vi "SIM_Drive_Gyro_EXECUTE.vi"(6 "FPGA_Time_Seconds":dbl, 8 "error in (no error)":errorcluster, 11 "ModuleStates":T1[](array[typedef]) {"Angle"."SIN" format="%13.4f"; "Angle"."COS" format="%13.4f"; "Angle"."VALUE" format="%13.4f"}) -> (0 "error out":errorcluster, 3 "GyroYawDegrees":dbl)   [LabVIEW 2023]
uses:
  <vilib>/Rock Robotics/WPI/ThirdParty/JAS_Junk/TrajLib/TypeDef/SWERVE_DRIVE_MODULE_STATE.ctl
  <vilib>/Rock Robotics/WPI/ThirdParty/JAS_Junk/TrajLib/TypeDef/ROTATION2D.ctl
  SIM_Drive_Globals.vi
  <vilib>/Rock Robotics/WPI/ThirdParty/JAS_Junk/TrajLib/Trajectory_Library.lvlib
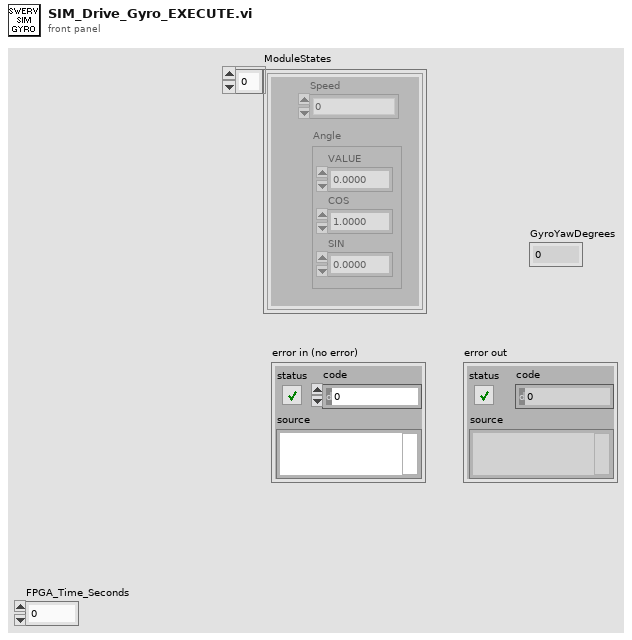
[diagram p1: front panel]
types:
  T1 = typedef "Trajectory_Library.lvlib/SWERVE_DRIVE_MODULE_STATE.ctl" = cluster{"Speed":dbl, "Angle":T2}
  T2 = typedef "Trajectory_Library.lvlib/ROTATION2D.ctl" = cluster{"VALUE":dbl, "COS":dbl, "SIN":dbl}
  T3 = typedef "Trajectory_Library.lvlib/SWERVE_DRIVE_KINEMATICS.ctl" = cluster{"NumModules":i32, "InverseKinematics":T4, "ForwardKinematics":T4, "Modules":T5[], "PrevCoR":T5, "SavedModuleStates":T1[]}
  T4 = typedef "NI_Matrix.lvlib/RealMatrix.ctl" = dbl[][]
  T5 = typedef "Trajectory_Library.lvlib/TRANSLATION2D.ctl" = cluster{"X":dbl, "Y":dbl}
  T6 = typedef "Trajectory_Library.lvlib/CHASSIS_SPEEDS.ctl" = cluster{"vX":dbl, "vY":dbl, "vOmega":dbl}
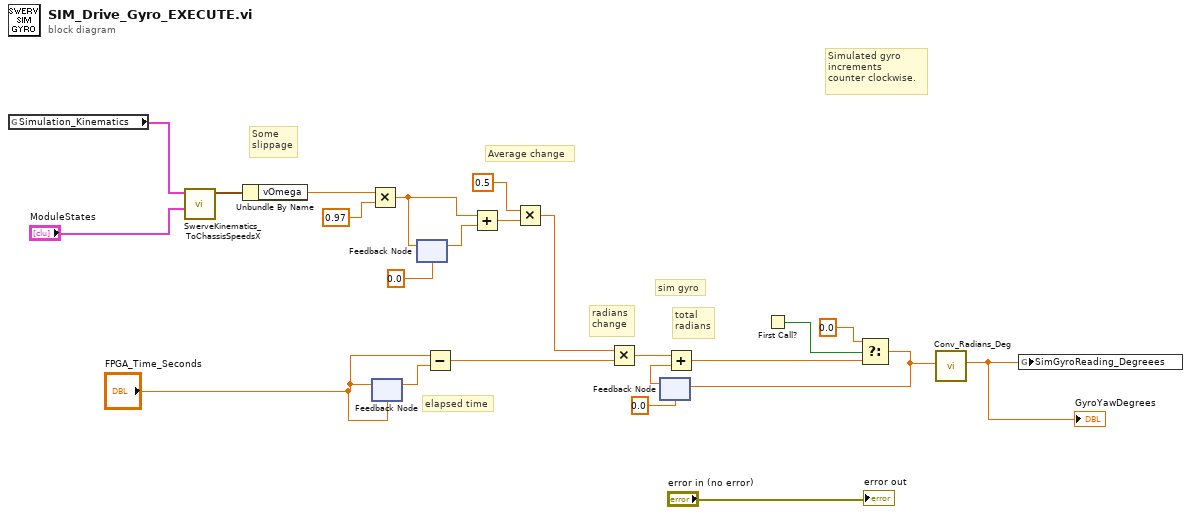
[diagram p0: block diagram]
diagram:
  # "Average change"
  # "Simulated gyro\nincrements\ncounter clockwise."
  # "Some \nslippage"
  # "elapsed time"
  # "total \nradians"
  # "radians \nchange"
  # "sim gyro"
  n1 = global read "SIM_Drive_Globals.vi" "Simulation_Kinematics"() -> (w6:T3)
  n2 = call <vilib>:"SwerveKinematics_ToChassisSpeedsX.vi"("WheelStates"="ModuleStates", "in SWERVE_DRIVE_KINEMATICS"=w6) -> ("Chassis Speed"=w7:T6)  [unwired: 9 in]
  n3 = Unbundle By Name(w7) -> ("vOmega"=w2:dbl)
  n4 = Multiply(x=w2, y=0.97) -> (x*y=w13:dbl)
  n5 = feedback #1("FPGA_Time_Seconds") -> (w20:dbl)
  n6 = feedback-in #1("FPGA_Time_Seconds") -> ()
  n7 = feedback-in #2(w13) -> ()
  n8 = feedback #2(0.0) -> (w12:dbl)
  n9 = Subtract(x="FPGA_Time_Seconds", y=w20) -> (x-y=w1:dbl)
  n10 = Add(x=w13, y=w12) -> (x+y=w10:dbl)
  n11 = Multiply(x=0.5, y=w10) -> (x*y=w8:dbl)
  n12 = Multiply(x=w8, y=w1) -> (x*y=w21:dbl)
  n13 = feedback #3(0.0) -> (w22:dbl)
  n14 = Add(x=w21, y=w22) -> (x+y=w5:dbl)
  n15 = First Call?() -> (First Call?: T/F=w3:bool)
  n16 = Select(t=0.0, s=w3, f=w5) -> (s? t:f=w15:dbl)
  n17 = feedback-in #3(w15) -> ()
  n18 = call <vilib>:"Conv_Radians_Deg.vi"("Radians"=w15) -> ("Degrees"=w18:dbl)  [unwired: 10 in]
  "GyroYawDegrees" <- w18
  n19 = global write "SIM_Drive_Globals.vi" "SimGyroReading_Degreees"(w18) -> ()
  "error out" <- "error in (no error)"
